vi "displayTriggeredStand.vi"(0 "Ch1 in":dbl[](array[numeric]), 1 "Ch2 in":dbl[](array[numeric]), 2 "threshold":dbl, 3 "Ch3 in":dbl[](array[numeric]), 4 "displayRange":i32, 5 "binning":i32=100, 6 "trigDisp (only square)":bool, 7 "Ch4 in":dbl[](array[numeric]), 8 "edgeStart":i32=100, 11 "VolTrig 3":dbl[][](array[numeric])) -> (12 "Ch1 out":dbl[](array[numeric]), 13 "VolTrig 2":dbl[](array[numeric]), 14 "Ch2 out":dbl[](array[numeric]), 15 "Ch3 out":dbl[](array[numeric]), 17 "Ch4 out":dbl[](array[numeric]), 18 "VolTrig":dbl[][](array[numeric]))   [LabVIEW 2021]
panel:
  out "size(s) 2":i32[](array[numeric])
  out "size(s)":i32[](array[numeric])
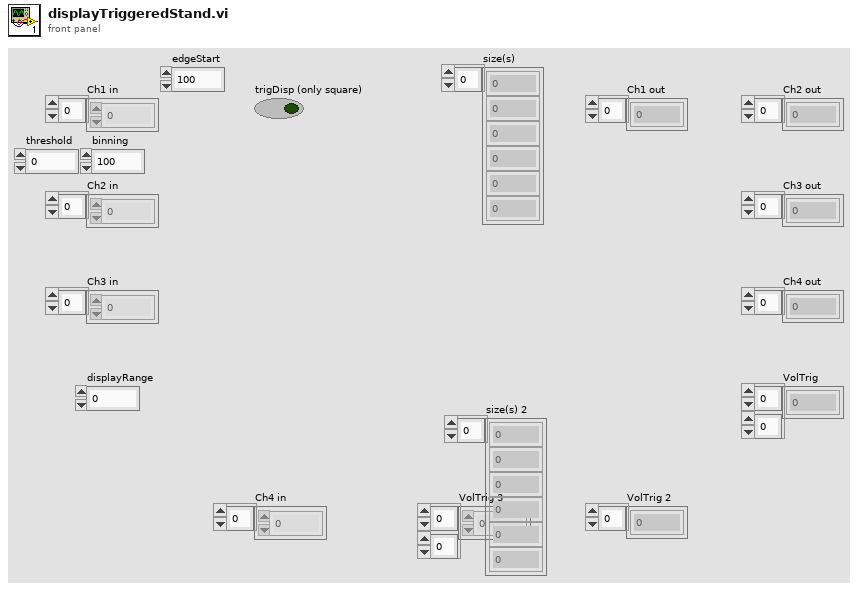
[diagram p1: front panel]
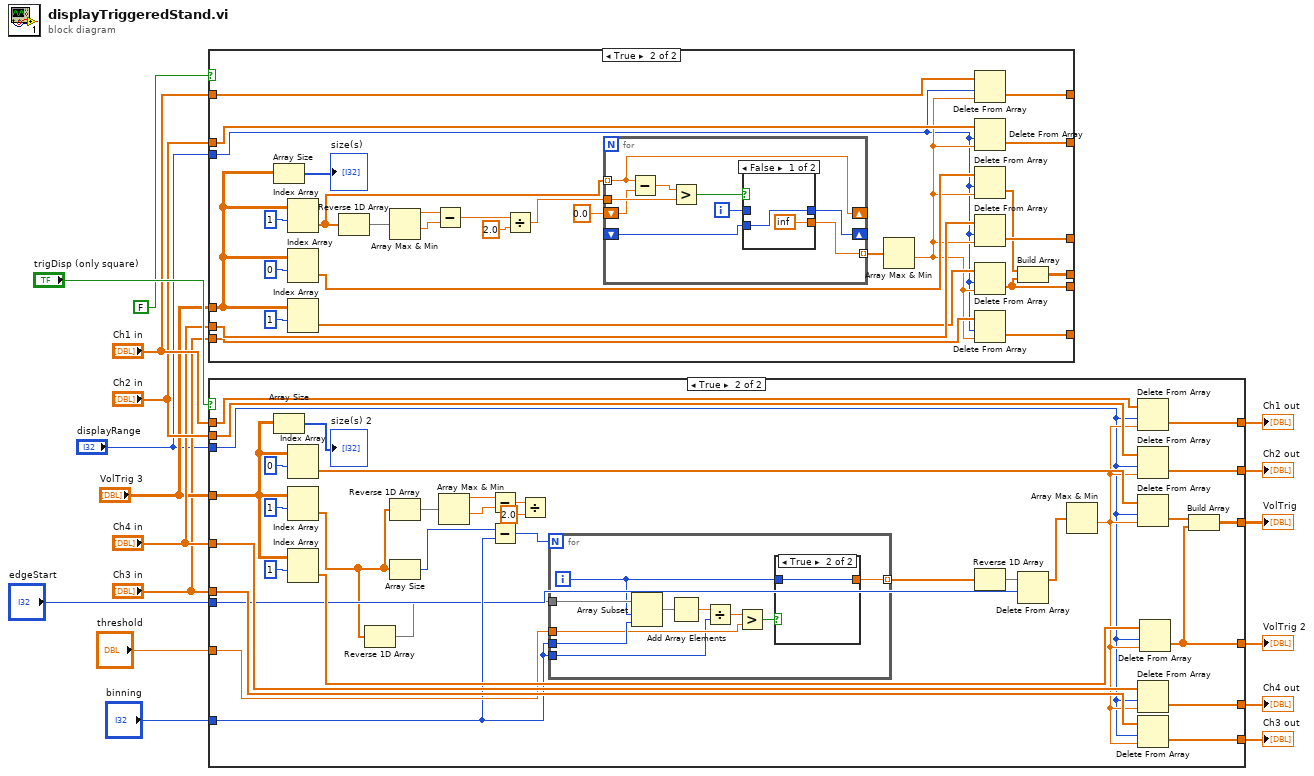
[diagram p0: block diagram]
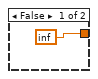
[diagram p3: hidden frame]
diagram:
  n1 = case shown="True" FALSE {
    tunnel: "displayRange" -> [_ w23]
    tunnel: "VolTrig 3" -> [w19 w26]
    tunnel: "Ch4 in" -> [w18 w42]
    tunnel: [w18 w41] -> _
    tunnel: "Ch3 in" -> [w22 w40]
    tunnel: [w22 w39] -> _
    tunnel: "Ch2 in" -> [w21 w38]
    tunnel: [w21 w37] -> _
    tunnel: "Ch1 in" -> [w20 w36]
    tunnel: [w20 w35] -> _
    tunnel: [w19 w27] -> _
    tunnel: [w18 w29] -> _
    frame False {
    }
    frame True {
      n2 = Array Size(array=w26) -> (size(s)=→"size(s)":i32[])
      n3 = Index Array(array=w26, index (row)=1) -> (element=w43:dbl[])  [unwired: 1 in]
      n4 = Index Array(array=w26, index (row)=0) -> (element=w31:dbl[])  [unwired: 1 in]
      n5 = Index Array(array=w26, index (row)=1) -> (element=w33:dbl[])  [unwired: 1 in]
      n6 = Reverse 1D Array(array=w43) -> (reversed array=w45:dbl[])
      n7 = Array Max & Min(array=w45) -> (max value=w51:dbl, min value=w50:dbl)  [unwired: 2 out]
      n8 = Subtract(x=w51, y=w50) -> (x-y=w49:dbl)
      n9 = Divide(x=w49, y=2.0) -> (x/y=w24:dbl)
      n10 = for {
        tunnel: w24 -> [w60]
        tunnel: w43 -> [w52] mode=indexing
        shift-right: [w52] -> _
        shift-left: 0.0 -> [w56]
        shift-right: [w57] -> _
        shift-left: _ -> [w54]
        tunnel: [w53] -> w46 mode=indexing
        i -> [w58]
        n11 = Subtract(x=w52, y=w56) -> (x-y=w55:dbl)
        n12 = Greater?(x=w55, y=w60) -> (0:w59:bool)
        n13 = case shown="False" w59 {
          tunnel: [w62 w63] -> w57
          tunnel: w58 -> [_ w63]
          tunnel: w54 -> [w62 _]
          tunnel: [inf w63] -> w53
          frame False {
          }
          frame True {
          }
        }
      }
      n14 = Array Max & Min(array=w46) -> (min value=w30:dbl)  [unwired: 3 out]
      n15 = Delete From Array(array=w36, length=w23, index=w30) -> (deleted portion=w35:dbl[])  [unwired: 1 out]
      n16 = Delete From Array(array=w38, length=w23, index=w30) -> (deleted portion=w37:dbl[])  [unwired: 1 out]
      n17 = Delete From Array(array=w31, length=w23, index=w30) -> (deleted portion=w28:dbl[])  [unwired: 1 out]
      n18 = Delete From Array(array=w42, length=w23, index=w30) -> (deleted portion=w41:dbl[])  [unwired: 1 out]
      n19 = Delete From Array(array=w33, length=w23, index=w30) -> (deleted portion=w29:dbl[])  [unwired: 1 out]
      n20 = Delete From Array(array=w40, length=w23, index=w30) -> (deleted portion=w39:dbl[])  [unwired: 1 out]
      n21 = Build Array(w28, w29) -> (w27:dbl[][])
    }
  }
  n22 = case shown="True" "trigDisp (only square)" {
    tunnel: "displayRange" -> [_ w80]
    tunnel: "VolTrig 3" -> [w65 w82]
    tunnel: "Ch4 in" -> [w64 w98]
    tunnel: [w64 w97] -> w7
    tunnel: "Ch3 in" -> [w68 w96]
    tunnel: [w68 w95] -> w5
    tunnel: "Ch2 in" -> [w67 w94]
    tunnel: [w67 w93] -> w9
    tunnel: "Ch1 in" -> [w66 w92]
    tunnel: [w66 w91] -> w10
    tunnel: [w65 w83] -> w8
    tunnel: [w64 w85] -> w6
    tunnel: "binning" -> [_ w75]
    tunnel: "threshold" -> [_ w79]
    tunnel: "edgeStart" -> [_ w71]
    frame False {
    }
    frame True {
      n23 = Array Size(array=w82) -> (size(s)=→"size(s) 2":i32[])
      n24 = Index Array(array=w82, index (row)=0) -> (element=w87:dbl[])  [unwired: 1 in]
      n25 = Index Array(array=w82, index (row)=1) -> (element=w70:dbl[])  [unwired: 1 in]
      n26 = Index Array(array=w82, index (row)=1) -> (element=w89:dbl[])  [unwired: 1 in]
      n27 = Reverse 1D Array(array=w70) -> (reversed array=w69:dbl[])
      n28 = Reverse 1D Array(array=w70) -> (reversed array=w76:dbl[])
      n29 = Array Size(array=w70) -> (size(s)=w78:i32)
      n30 = Array Max & Min(array=w76) -> (max value=w103:dbl, min value=w102:dbl)  [unwired: 2 out]
      n31 = Subtract(x=w103, y=w102) -> (x-y=w101:dbl)
      n32 = Subtract(x=w78, y=w75) -> (x-y=w77:i32)
      n33 = Divide(x=w101, y=2.0) -> ()  [unwired: 1 out]
      n34 = for {
        N: w77 -> [_]
        tunnel: [w113] -> w73 mode=indexing
        tunnel: w69 -> [w112]
        tunnel: w75 -> [w110]
        tunnel: w79 -> [w108]
        tunnel: w75 -> [w104]
        i -> [w111]
        n35 = Array Subset(array=w112, index=w111, length=w110) -> (w109:dbl[])
        n36 = Add Array Elements(numeric array=w109) -> (sum=w105:dbl)
        n37 = Divide(x=w105, y=w104) -> (x/y=w106:dbl)
        n38 = Greater?(x=w106, y=w108) -> (0:w107:bool)
        n39 = case shown="True" w107 {
          tunnel: w111 -> [_ w115]
          tunnel: [inf w115] -> w113
          frame False {
          }
          frame True {
          }
        }
      }
      n40 = Reverse 1D Array(array=w73) -> (reversed array=w72:dbl[])
      n41 = Delete From Array(array=w72, length=w71) -> (array with subset deleted=w74:dbl[])  [unwired: 1 in, 1 out]
      n42 = Array Max & Min(array=w74) -> (min value=w86:dbl)  [unwired: 3 out]
      n43 = Delete From Array(array=w92, length=w80, index=w86) -> (deleted portion=w91:dbl[])  [unwired: 1 out]
      n44 = Delete From Array(array=w94, length=w80, index=w86) -> (deleted portion=w93:dbl[])  [unwired: 1 out]
      n45 = Delete From Array(array=w87, length=w80, index=w86) -> (deleted portion=w84:dbl[])  [unwired: 1 out]
      n46 = Delete From Array(array=w98, length=w80, index=w86) -> (deleted portion=w97:dbl[])  [unwired: 1 out]
      n47 = Delete From Array(array=w96, length=w80, index=w86) -> (deleted portion=w95:dbl[])  [unwired: 1 out]
      n48 = Delete From Array(array=w89, length=w80, index=w86) -> (deleted portion=w85:dbl[])  [unwired: 1 out]
      n49 = Build Array(w84, w85) -> (w83:dbl[][])
    }
  }
  "VolTrig" <- w8
  "VolTrig 2" <- w6
  "Ch1 out" <- w10
  "Ch2 out" <- w9
  "Ch3 out" <- w5
  "Ch4 out" <- w7
